vi "RT Loop - System Health and FPGA Monitoring.vi"(11 "Message Queue":refnum<queue>) -> ()   [LabVIEW 2018]
uses:
  support/Message Queue/Message Cluster.ctl
  controls/FPGA VI Reference.ctl
  Globals/Global - Configuration Options.vi
  Globals/Global - All RT Loop Stop.vi
  Globals/Global - Monitoring Variables.vi
  <vilib>/Utility/error.llb/Error Cluster From Error Code.vi
  <vilib>/rvi/errors/niLvFpgaAdjustHostInterfaceError.vi
  <vilib>/nisyscfg/Close (System).vi
  <vilib>/rvi/interface/nirviReadWriteControl/nirviReadWriteControl.xnode
  <vilib>/NI_Real-Time Target Support.lvlib
  <vilib>/nisyscfg/nisyscfg.lvlib
  <resource>/objmgr/nisysapi.rc
  NiFpgaLv.dll
  <vilib>/rvi/interface/Simulation/niFpgaSimulationCallBeginRW.vi
  support/Message Queue/Message Queue.lvlib
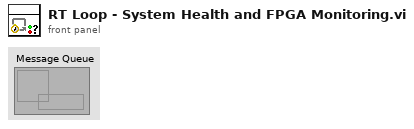
[diagram p1: front panel]
types:
  T1 = typedef "FPGA VI Reference.ctl" = refnum<k20>
  T2 = typedef "NI_Real-Time Target Support.lvlib/RT CPU Load.ctl" = cluster{"Total (%)":dbl, "Time Critical (%)":dbl, "Timed Structures (%)":dbl, "High (%)":dbl, "Above Normal (%)":dbl, "Normal (%)":dbl, "Background (%)":dbl, "Idle (%)":dbl, "ISR (%)":dbl}
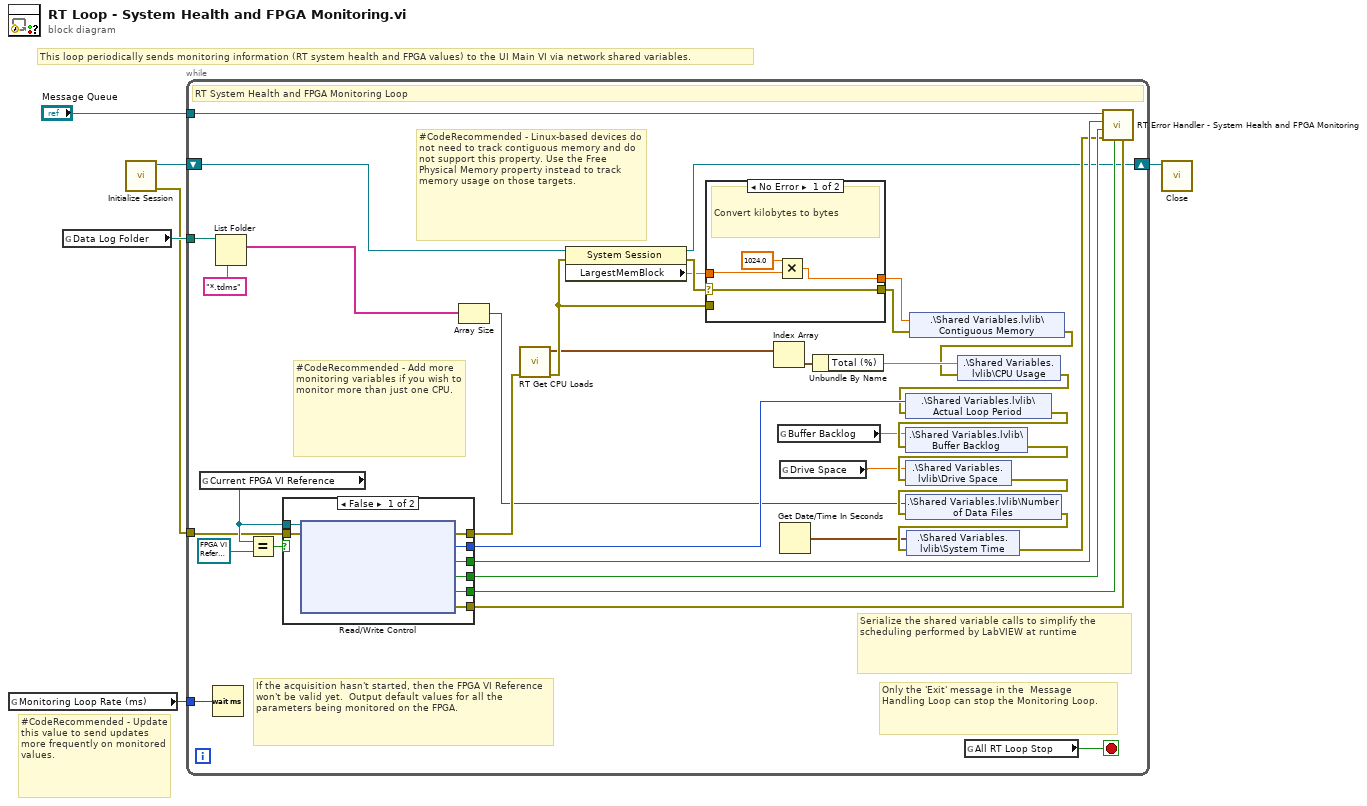
[diagram p0: block diagram]
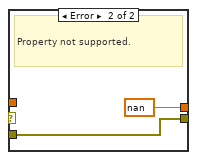
[diagram p2: hidden frame]
diagram:
  # "#CodeRecommended - Update this value to send updates more frequently on monitored values."
  # "This loop periodically sends monitoring information (RT system health and FPGA values) to the UI Main VI via network shared variables."
  n1 = global read "Global - Configuration Options.vi" "Monitoring Loop Rate (ms)"() -> (w5:u32)
  n2 = global read "Global - Configuration Options.vi" "Data Log Folder"() -> (w4:path)
  n3 = call <vilib>:"Initialize Session.vi"() -> ("error out"=w1:errorcluster, "Session out"=w3:refnum<k21>)  [unwired: 10 in]
  n4 = while {
    tunnel: "Message Queue" -> [w38]
    tunnel: w5 -> [w37]
    tunnel: w4 -> [w21]
    shift-right: [w13] -> w2
    shift-left: w3 -> [w14]
    tunnel: w1 -> [w10]
    stop <- w39 stop-if-true
    # "#CodeRecommended - Linux-based devices do not need to track contiguous memory and do not support this property. Use the Free Physical Memory property instead to track memory usage on those targets."
    # "#CodeRecommended - Add more monitoring variables if you wish to monitor more than just one CPU."
    # "If the acquisition hasn't started, then the FPGA VI Reference won't be valid yet.  Output default values for all the parameters being monitored on the FPGA."
    # "Serialize the shared variable calls to simplify the scheduling performed by LabVIEW at runtime"
    # "Only the 'Exit' message in the  Message Handling Loop can stop the Monitoring Loop."
    # "RT System Health and FPGA Monitoring Loop"
    n5 = global read "Global - Monitoring Variables.vi" "Current FPGA VI Reference"() -> (w28:T1)
    n6 = Wait (ms)(milliseconds to wait=w37) -> ()  [unwired: 1 out]
    n7 = List Folder(path=w21, pattern="*.tdms") -> (filenames=w19:string[])  [unwired: 2 in, 3 out]
    n8 = Equal?(x=w28, y=T1 refnum ("Current FPGA VI Reference")) -> (x = y?=w26:bool)
    n9 = case shown="False" w26 {
      tunnel: [w57 _] -> w36
      tunnel: [w56 _] -> w35
      tunnel: [w55 _] -> w34
      tunnel: [w54 _] -> w33
      tunnel: [w53 _] -> w32
      tunnel: [w52 _] -> w31
      tunnel: w28 -> [w51 _]
      tunnel: w10 -> [w50 _]
      frame False {
        n10 = xnode "Read/Write Control"("FPGA VI Reference In"=w51, "error in"=w50) -> ("error out"=w57:errorcluster, "Actual Loop Period (ticks)"=w56:u32, "Module Underflow"=w55:bool, "DMA FIFO Full"=w54:bool, "Different Channel Count"=w53:bool, "FPGA Error"=w52:errorcluster)  [unwired: 1 out]
      }
      frame True {
      }
    }
    n11 = Array Size(array=w19) -> (size(s)=w18:i32)
    n12 = call <vilib>:"RT Get CPU Loads.vi"("error in (no error)"=w36) -> ("error out"=w43:errorcluster, "CPU loads"=w41:T2[])  [unwired: 9 in]
    n13 = property class="System Session"(reference=w14, error in=w43) -> (reference out=w13:refnum<k21>, error out=w42:errorcluster, "LargestMemBlock"=w7:dbl)
    n14 = case shown="No Error" w42 {
      selector: w42 -> [w44 _]
      tunnel: w7 -> [w46 _]
      tunnel: [w45 nan] -> w9
      tunnel: [w44 w48] -> w8
      tunnel: w43 -> [_ w48]
      frame No Error {
        # "Convert kilobytes to bytes"
        n15 = Multiply(x=1024.0, y=w46) -> (x*y=w45:dbl)
      }
      frame Error {
        # "Property not supported."
      }
    }
    n16 = Index Array(array=w41) -> (element=w40:T2)  [unwired: 1 in]
    n17 = global read "Global - Monitoring Variables.vi" "Buffer Backlog"() -> (w29:dbl)
    n18 = global read "Global - Monitoring Variables.vi" "Drive Space"() -> (w23:dbl)
    n19 = Get Date/Time In Seconds() -> (seconds since 1Jan1904=w15:timestamp)
    n20 = Unbundle By Name(w40) -> ("Total (%)"=w25:dbl)
    n21 = shared-variable ".\\Shared Variables.lvlib\\Contiguous Memory"(w9, error in=w8) -> (error out=w12:errorcluster)
    n22 = shared-variable ".\\Shared Variables.lvlib\\CPU Usage"(w25, error in=w12) -> (error out=w11:errorcluster)
    n23 = shared-variable ".\\Shared Variables.lvlib\\Actual Loop Period"(w35, error in=w11) -> (error out=w30:errorcluster)
    n24 = shared-variable ".\\Shared Variables.lvlib\\Buffer Backlog"(w29, error in=w30) -> (error out=w24:errorcluster)
    n25 = shared-variable ".\\Shared Variables.lvlib\\Drive Space"(w23, error in=w24) -> (error out=w22:errorcluster)
    n26 = shared-variable ".\\Shared Variables.lvlib\\Number of Data Files"(w18, error in=w22) -> (error out=w17:errorcluster)
    n27 = shared-variable ".\\Shared Variables.lvlib\\System Time"(w15, error in=w17) -> (error out=w16:errorcluster)
    n28 = global read "Global - All RT Loop Stop.vi" "All RT Loop Stop"() -> (w39:bool)
    n29 = call "RT Error Handler - System Health and FPGA Monitoring.vi"("FPGA Error (FPGA)"=w31, "Different Channel Count (FPGA)"=w32, "error in (no error)"=w16, "DMA FIFO Full (FPGA)"=w33, "Module Underflow (FPGA)"=w34, "Message Queue"=w38) -> ()  [unwired: 5 in, 1 out]
  }
  n30 = call-poly <vilib>:"Close.vi"("Session in"=w2) -> ()  [unwired: 10 in, 1 out]
